vi "Taiko_Taglist.vi"() -> ()   [LabVIEW 2017]
uses:
  _lib/PDLM/pdlm_lib_x86_x64_UIThread.llb/PDLM_TaggedValueList.ctl
  _lib/PDLM/pdlm_lib_x86_x64_UIThread.llb/PDLM_TaggedValue.ctl
  _lib/PDLM/pdlm_lib_x86_x64_UIThread.llb/PDLM_Tag.ctl
panel:
  out "String out":string
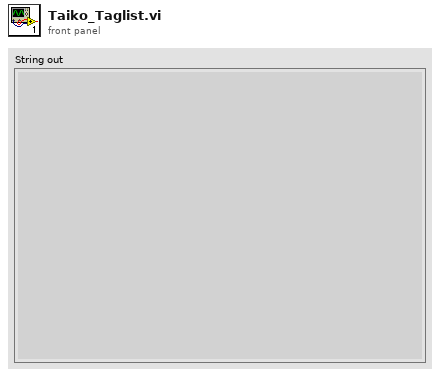
[diagram p1: front panel]
types:
  T1 = typedef "PDLM_TaggedValueList.ctl" = T2[]
  T2 = typedef "PDLM_TaggedValue.ctl" = cluster{"Tag":T3, "Value":u32}
  T3 = typedef "PDLM_Tag.ctl" = u32
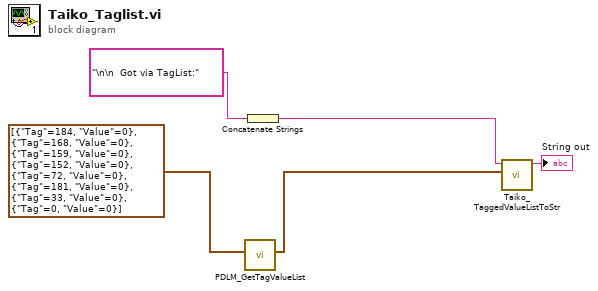
[diagram p0: block diagram]
diagram:
  n1 = call "PDLM_GetTagValueList.vi"("TaggedValueList"=T1 [{"Tag"=184, "Value"=0}, {"Tag"=168, "Value"=0}, {"Tag"=159, "Value"=0}, {"Tag"=152, "Value"=0}, {"Tag"=72, "Value"=0}, {"Tag"=181, "Value"=0}, {"Tag"=33, "Value"=0}, {"Tag"=0, "Value"=0}]) -> ("TaggedValueList out"=w4:T1)  [unwired: 8 in, 2 out]
  n2 = Concatenate Strings("\n\n  Got via TagList:" ("string")) -> (w3:string)
  n3 = call "Taiko_TaggedValueListToStr.vi"("TaggedValueList in"=w4, "String in"=w3) -> ("String out"=→"String out":string)  [unwired: 9 in]
